vi "Binary Config without Class Unit Tests.vi"(8 "error in (no error)":errorcluster) -> (0 "error out":errorcluster)   [LabVIEW 2021]
uses:
  Source/Constants/Support/Bool/Const_Bool.lvclass
  C:/New folder/LV_Abstract/LV_Abstract/Source/Abs_Types/Type/Abs_Type.lvclass
  C:/New folder/LV_Abstract/LV_Abstract/Source/Abs_Types/Boolean/Abs_Boolean.lvclass
  Source/Constants/Support/Str/Const_Str.lvclass
  C:/New folder/LV_Abstract/LV_Abstract/Source/Abs_Types/String/Abs_String.lvclass
  Source/Constants/Support/Time/Const_Time.lvclass
  C:/New folder/LV_Abstract/LV_Abstract/Source/Abs_Types/Time/Abs_Time.lvclass
  Source/Constants/Support/DBL/Const_DBL.lvclass
  C:/New folder/LV_Abstract/LV_Abstract/Source/Abs_Types/Double Float/Abs_Double Float.lvclass
  Source/Constants/Support/EXT/Const_EXT.lvclass
  C:/New folder/LV_Abstract/LV_Abstract/Source/Abs_Types/Extended Float/Abs_Extended Float.lvclass
  Source/Constants/Support/SGL/Const_SGL.lvclass
  C:/New folder/LV_Abstract/LV_Abstract/Source/Abs_Types/Single Float/Abs_Single Float.lvclass
  Source/Constants/Support/CPLX_DBL/Const_CPLX_DBL.lvclass
  C:/New folder/LV_Abstract/LV_Abstract/Source/Abs_Types/Complex Double Float/Abs_Complex Double Float.lvclass
  Source/Constants/Support/CPLX_EXT/Const_CPLX_EXT.lvclass
  C:/New folder/LV_Abstract/LV_Abstract/Source/Abs_Types/Complex Extended Float/Abs_Complex Extended Float.lvclass
  Source/Constants/Support/CPLX_SGL/Const_CPLX_SGL.lvclass
  C:/New folder/LV_Abstract/LV_Abstract/Source/Abs_Types/Complex Single Float/Abs_Complex Single Float.lvclass
  Source/Constants/Support/I8/Const_I8.lvclass
  C:/New folder/LV_Abstract/LV_Abstract/Source/Abs_Types/I8 Integer/Abs_I8 Integer.lvclass
  Source/Constants/Support/I16/Const_I16.lvclass
  C:/New folder/LV_Abstract/LV_Abstract/Source/Abs_Types/I16 Integer/Abs_I16 Integer.lvclass
  Source/Constants/Support/I32/Const_I32.lvclass
  C:/New folder/LV_Abstract/LV_Abstract/Source/Abs_Types/I32 Integer/Abs_I32 Integer.lvclass
  Source/Constants/Support/I64/Const_I64.lvclass
  C:/New folder/LV_Abstract/LV_Abstract/Source/Abs_Types/I64 Integer/Abs_I64 Integer.lvclass
  Source/Constants/Support/U8/Const_U8.lvclass
  C:/New folder/LV_Abstract/LV_Abstract/Source/Abs_Types/U8 Integer/Abs_U8 Integer.lvclass
  Source/Constants/Support/U16/Const_U16.lvclass
  C:/New folder/LV_Abstract/LV_Abstract/Source/Abs_Types/U16 Integer/Abs_U16 Integer.lvclass
  Source/Constants/Support/U32/Const_U32.lvclass
  C:/New folder/LV_Abstract/LV_Abstract/Source/Abs_Types/U32 Integer/Abs_U32 Integer.lvclass
  Source/Constants/Support/U64/Const_U64.lvclass
  C:/New folder/LV_Abstract/LV_Abstract/Source/Abs_Types/U64 Integer/Abs_U64 Integer.lvclass
  02b2badb-acca-4382-accc-9e0cbca89e75.vi
  3a5694f5-013d-4b07-84b6-ea3c9536ba0f.vi
  2b2927a9-8b8c-48da-98b9-aa801b3b90f6.vi
  49527974-12a0-4c80-8f50-9a472cb1ac6a.vi
  f2baf64f-1945-416f-b3e1-cbab6fa2e840.vi
  854b162c-b87d-448f-bcf5-e18436ea6453.vi
  7c8ea99b-82f2-4f54-b01f-3f412c8ffb04.vi
  5f0fb255-70b7-420f-a810-2646098efdc7.vi
  00c9cc81-24da-46d5-8c2d-29c94b341ce8.vi
  a708557e-5d5b-43c6-97ed-bafcd6ec96b3.vi
  f4c84a6e-e62e-4878-8cb8-6a34f8140e46.vi
  20f0a36a-91be-4dca-b05a-48252f72b155.vi
  4e9ae80b-1b7d-4b59-a33c-58db0d6d6edd.vi
  e86d4e46-72b0-48cb-a17e-7d580fcd9531.vi
  1f3f42c3-23d4-4482-8cf7-40cf6075775f.vi
  b5e941fb-31ab-4b34-bd06-624bd25f61f3.vi
  e94631f0-9f0e-4e5e-b1c8-b18dcdbd6442.vi
  Source/Abs_Types/Abs_Simple_Read.vi
  Source/Abs_Types/Boolean/Simple Read.vi
  Source/Abs_Types/String/Simple Read.vi
  Source/Abs_Types/Time/Simple Read.vi
  Source/Abs_Types/Double Float/Simple Read.vi
  Source/Abs_Types/Extended Float/Simple Read.vi
  Source/Abs_Types/Single Float/Simple Read.vi
  Source/Abs_Types/I8 Integer/Simple Read.vi
  Source/Abs_Types/I16 Integer/Simple Read.vi
  Source/Abs_Types/I32 Integer/Simple Read.vi
  Source/Abs_Types/I64 Integer/Simple Read.vi
  Source/Abs_Types/U8 Integer/Simple Read.vi
  Source/Abs_Types/U16 Integer/Simple Read.vi
  Source/Abs_Types/U32 Integer/Simple Read.vi
  Source/Abs_Types/U64 Integer/Simple Read.vi
  <vilib>/Utility/Data Type/Get Type Information.vi
  Source/Constants/Abs_Constant.vi
  Source/Constants/Support/Bool/Bool.vi
  <vilib>/addons/_JKI Toolkits/Caraya/classes/Test/Define Test.vi
  Source/Abs_Types/Type/Read Config Binary.vi
  <vilib>/addons/_JKI Toolkits/Caraya/classes/Assert/Assert.vi
  <vilib>/addons/_JKI Toolkits/Caraya/classes/Assert/Assert Equal Value_Variant.vi
  <vilib>/addons/_JKI Toolkits/Caraya/classes/Assert/Assert Equal Type_Variant.vi
  Source/Constants/Support/Str/Str.vi
  Source/Constants/Support/Time/Time.vi
  Source/Constants/Support/DBL/DBL.vi
  Source/Constants/Support/EXT/EXT.vi
  Source/Constants/Support/SGL/SGL.vi
  Source/Constants/Support/CPLX_DBL/CPLX_DBL.vi
  Source/Abs_Types/Complex Double Float/Simple Read.vi
  Source/Constants/Support/CPLX_EXT/CPLX_EXT.vi
  Source/Abs_Types/Complex Extended Float/Simple Read.vi
  Source/Constants/Support/CPLX_SGL/CPLX_SGL.vi
  Source/Abs_Types/Complex Single Float/Simple Read.vi
  Source/Constants/Support/I8/I8.vi
  Source/Constants/Support/I16/I16.vi
  Source/Constants/Support/I32/I32.vi
  Source/Constants/Support/I64/I64.vi
  Source/Constants/Support/U8/U8.vi
  Source/Constants/Support/U16/U16.vi
  Source/Constants/Support/U32/U32.vi
  Source/Constants/Support/U64/U64.vi
  Source/Abs_Types/Boolean/Abs_Boolean.lvclass
  Source/Abs_Types/String/Abs_String.lvclass
  Source/Abs_Types/Time/Abs_Time.lvclass
  Source/Abs_Types/Double Float/Abs_Double Float.lvclass
  Source/Abs_Types/Extended Float/Abs_Extended Float.lvclass
  Source/Abs_Types/Single Float/Abs_Single Float.lvclass
  Source/Abs_Types/Complex Double Float/Abs_Complex Double Float.lvclass
  Source/Abs_Types/Complex Extended Float/Abs_Complex Extended Float.lvclass
  Source/Abs_Types/Complex Single Float/Abs_Complex Single Float.lvclass
  Source/Abs_Types/I8 Integer/Abs_I8 Integer.lvclass
  Source/Abs_Types/I16 Integer/Abs_I16 Integer.lvclass
  Source/Abs_Types/I32 Integer/Abs_I32 Integer.lvclass
  Source/Abs_Types/I64 Integer/Abs_I64 Integer.lvclass
  Source/Abs_Types/U8 Integer/Abs_U8 Integer.lvclass
  Source/Abs_Types/U16 Integer/Abs_U16 Integer.lvclass
  Source/Abs_Types/U32 Integer/Abs_U32 Integer.lvclass
  Source/Abs_Types/U64 Integer/Abs_U64 Integer.lvclass
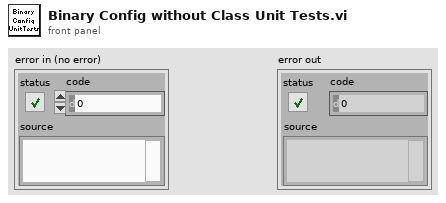
[diagram p1: front panel]
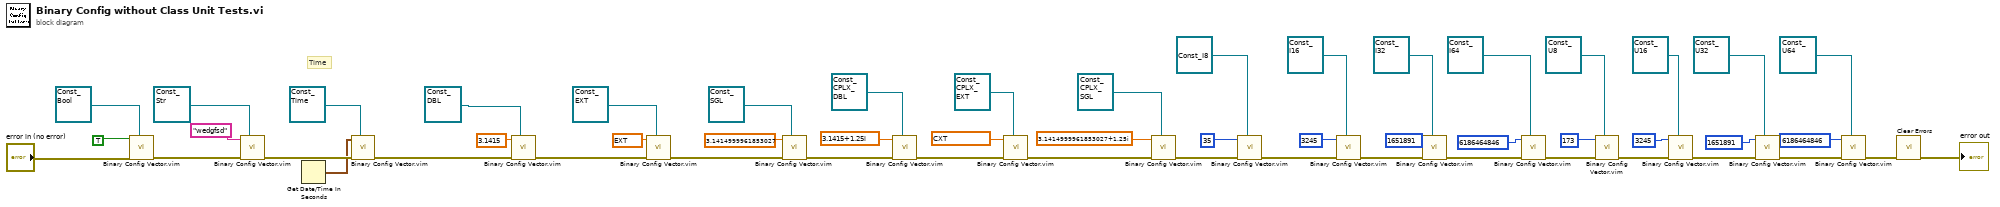
[diagram p0: block diagram]
diagram:
  # "Time"
  n1 = call "Binary Config Vector.vim"("Expected Class"=refnum<class "Const_Bool.lvclass"> refnum ("Const_Bool.lvclass"), "error in (no error)"="error in (no error)", "Test Value"=TRUE) -> ("error out"=w46:errorcluster)  [unwired: 8 in]
  n2 = call "Binary Config Vector.vim"("Expected Class"=refnum<class "Const_Str.lvclass"> refnum ("Const_Str.lvclass"), "error in (no error)"=w46, "Test Value"="wedgfsd") -> ("error out"=w45:errorcluster)  [unwired: 8 in]
  n3 = Get Date/Time In Seconds() -> (seconds since 1Jan1904=w43:timestamp)
  n4 = call "Binary Config Vector.vim"("Expected Class"=refnum<class "Const_Time.lvclass"> refnum ("Const_Time.lvclass"), "error in (no error)"=w45, "Test Value"=w43) -> ("error out"=w44:errorcluster)  [unwired: 8 in]
  n5 = call "Binary Config Vector.vim"("Expected Class"=refnum<class "Const_DBL.lvclass"> refnum ("Const_DBL.lvclass"), "error in (no error)"=w44, "Test Value"=3.1415) -> ("error out"=w51:errorcluster)  [unwired: 8 in]
  n6 = call "Binary Config Vector.vim"("Expected Class"=refnum<class "Const_EXT.lvclass"> refnum ("Const_EXT.lvclass"), "error in (no error)"=w51, "Test Value"=ext 3.1414999999999999999) -> ("error out"=w48:errorcluster)  [unwired: 8 in]
  n7 = call "Binary Config Vector.vim"("Expected Class"=refnum<class "Const_SGL.lvclass"> refnum ("Const_SGL.lvclass"), "error in (no error)"=w48, "Test Value"=sgl 3.1415) -> ("error out"=w42:errorcluster)  [unwired: 8 in]
  n8 = call "Binary Config Vector.vim"("Expected Class"=refnum<class "Const_CPLX_DBL.lvclass"> refnum ("Const_CPLX_DBL.lvclass"), "error in (no error)"=w42, "Test Value"=cdb 3.1415+1.25i) -> ("error out"=w39:errorcluster)  [unwired: 8 in]
  n9 = call "Binary Config Vector.vim"("Expected Class"=refnum<class "Const_CPLX_EXT.lvclass"> refnum ("Const_CPLX_EXT.lvclass"), "error in (no error)"=w39, "Test Value"=cxt 3.1415+1.25i) -> ("error out"=w37:errorcluster)  [unwired: 8 in]
  n10 = call "Binary Config Vector.vim"("Expected Class"=refnum<class "Const_CPLX_SGL.lvclass"> refnum ("Const_CPLX_SGL.lvclass"), "error in (no error)"=w37, "Test Value"=csg 3.1415+1.25i) -> ("error out"=w36:errorcluster)  [unwired: 8 in]
  n11 = call "Binary Config Vector.vim"("Expected Class"=refnum<class "Const_I8.lvclass"> refnum ("Const_I8.lvclass"), "error in (no error)"=w36, "Test Value"=i8 35) -> ("error out"=w33:errorcluster)  [unwired: 8 in]
  n12 = call "Binary Config Vector.vim"("Expected Class"=refnum<class "Const_I16.lvclass"> refnum ("Const_I16.lvclass"), "error in (no error)"=w33, "Test Value"=i16 3245) -> ("error out"=w31:errorcluster)  [unwired: 8 in]
  n13 = call "Binary Config Vector.vim"("Expected Class"=refnum<class "Const_I32.lvclass"> refnum ("Const_I32.lvclass"), "error in (no error)"=w31, "Test Value"=1651891) -> ("error out"=w30:errorcluster)  [unwired: 8 in]
  n14 = call "Binary Config Vector.vim"("Expected Class"=refnum<class "Const_I64.lvclass"> refnum ("Const_I64.lvclass"), "error in (no error)"=w30, "Test Value"=i64 6186464846) -> ("error out"=w27:errorcluster)  [unwired: 8 in]
  n15 = call "Binary Config Vector.vim"("Expected Class"=refnum<class "Const_U8.lvclass"> refnum ("Const_U8.lvclass"), "error in (no error)"=w27, "Test Value"=u8 173) -> ("error out"=w26:errorcluster)  [unwired: 8 in]
  n16 = call "Binary Config Vector.vim"("Expected Class"=refnum<class "Const_U16.lvclass"> refnum ("Const_U16.lvclass"), "error in (no error)"=w26, "Test Value"=u16 3245) -> ("error out"=w24:errorcluster)  [unwired: 8 in]
  n17 = call "Binary Config Vector.vim"("Expected Class"=refnum<class "Const_U32.lvclass"> refnum ("Const_U32.lvclass"), "error in (no error)"=w24, "Test Value"=u32 1651891) -> ("error out"=w22:errorcluster)  [unwired: 8 in]
  n18 = call "Binary Config Vector.vim"("Expected Class"=refnum<class "Const_U64.lvclass"> refnum ("Const_U64.lvclass"), "error in (no error)"=w22, "Test Value"=u64 6186464846) -> ("error out"=w20:errorcluster)  [unwired: 8 in]
  n19 = call <vilib>:"Clear Errors.vi"("error in (no error)"=w20) -> ("error out"=→"error out":errorcluster)  [unwired: 5 in, 1 out]
